vi "Send_UIVisibleCtrlArray.vi"(8 "error in":errorcluster, 9 "Visible":bool[](array[boolean]), 10 "Control Label":string[](array[string]), 11 "Queue in":refnum<queue>) -> (0 "error out":errorcluster)   [LabVIEW 2018, in "UI_Library.lvlib"]
uses:
  UI_Library.lvlib
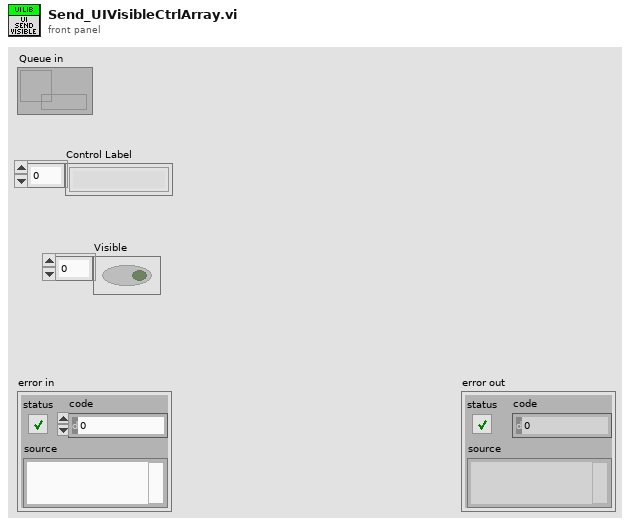
[diagram p1: front panel]
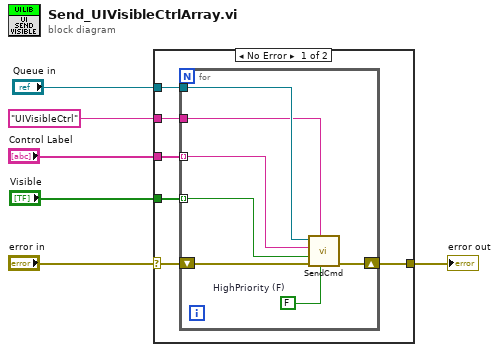
[diagram p0: block diagram]
diagram:
  n1 = case shown="No Error" "error in" {
    selector: "error in" -> [w11 w20]
    tunnel: "Queue in" -> [w12 _]
    tunnel: "Control Label" -> [w8 _]
    tunnel: "Visible" -> [w7 _]
    tunnel: "UIVisibleCtrl" ("UICmd") -> [w9 _]
    tunnel: [w10 w20] -> w6
    frame No Error {
      n2 = for {
        tunnel: w12 -> [w19]
        tunnel: w9 -> [w16]
        tunnel: w8 -> [w15] mode=indexing
        tunnel: w7 -> [w14] mode=indexing
        shift-right: [w17] -> w10
        shift-left: w11 -> [w18]
        w13 = FALSE  # HighPriority (F)
        n3 = call "SendCmd.vi"("HighPriority (F)"=w13, "UICmd"=w16, "error in"=w18, "Control Data"=w14, "Control Label"=w15, "Queue in"=w19) -> ("error out"=w17:errorcluster)  [unwired: 5 in]
      }
    }
    frame Error {
    }
  }
  "error out" <- w6
